vi "FT_Reset_Device.vi"(1 "Handle":u32) -> (0 "FT_Status":u32)   [LabVIEW 2013]
uses:
  FTD2XX.dll
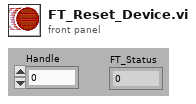
[diagram p1: front panel]
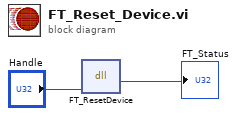
[diagram p0: block diagram]
diagram:
  n1 = dll-call lib="FTD2XX.dll" fn="FT_ResetDevice"("Handle"="Handle") -> ("FT_Status"=→"FT_Status":u32)  [unwired: 4 in, 2 out]
